vi "Signal Loop.vi"(8 "error in (no error)":errorcluster, 11 "CLI in":refnum<class "CLI.lvclass">) -> (0 "error out":errorcluster)   [LabVIEW 2017, in "CLI.lvclass"]
uses:
  CLI.lvclass
  CLI.lvclass/CLI.ctl
panel:
  # "Connector Pane"
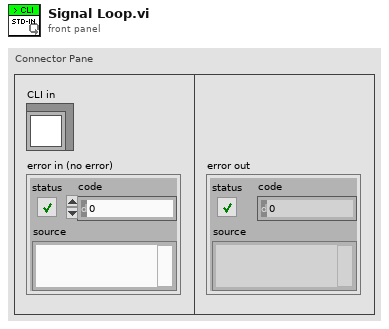
[diagram p1: front panel]
types:
  T1 = typedef "Events.ctl" = cluster{"STIN":refnum<user-event>, "SIGI":refnum<user-event>, "UnknownSignal":refnum<user-event>}
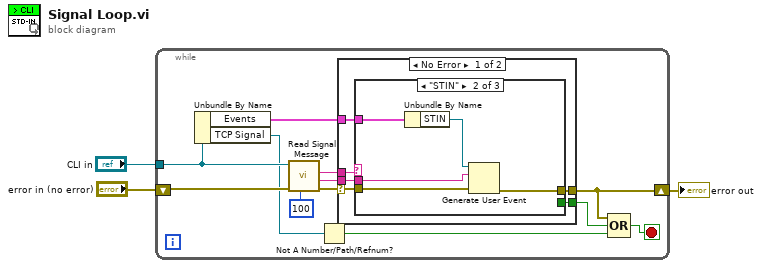
[diagram p0: block diagram]
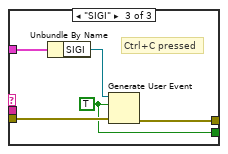
[diagram p3: hidden frame]
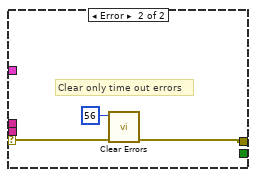
[diagram p4: hidden frame]
diagram:
  n1 = while {
    tunnel: "CLI in" -> [w10]
    shift-right: [w5] -> w1
    shift-left: "error in (no error)" -> [w15]
    stop <- w11 stop-if-true
    n2 = Unbundle By Name(w10) -> ("Events"=w7:T1, "TCP Signal"=w9:refnum<k5>)
    n3 = call "Read Signal Message.vi"("timeout ms (25000)"=100, "error in (no error)"=w15, "CLI in"=w10) -> ("error out"=w12:errorcluster, "Message Contents"=w13:string, "Message Type"=w14:string)  [unwired: 5 in, 1 out]
    n4 = Not A Number/Path/Refnum?(number/path/refnum=w9) -> (NaN/Path/Refnum?=w8:bool)
    n5 = case shown="No Error" w12 {
      selector: w12 -> [w19 w35]
      tunnel: w14 -> [w21 _]
      tunnel: w13 -> [w20 _]
      tunnel: w7 -> [w18 _]
      tunnel: [w17 w34] -> w5
      tunnel: [w16 _] -> w4
      frame No Error {
        n6 = case shown="\"STIN\"" w21 {
          tunnel: w18 -> [_ w23 w29]
          tunnel: w20 -> [_ w26 _]
          tunnel: w19 -> [w22 w25 w31]
          tunnel: [w22 w24 w30] -> w17
          tunnel: [_ _ w28] -> w16
          frame Default {
          }
          frame "STIN" {
            n7 = Unbundle By Name(w23) -> ("STIN"=w27:refnum<user-event>)
            n8 = Generate User Event(user event=w27, event data cluster=w26, error in=w25) -> (error out=w24:errorcluster)  [unwired: 1 in, 1 out]
          }
          frame "SIGI" {
            w28 = TRUE ("event data")
            # "Ctrl+C pressed"
            n9 = Unbundle By Name(w29) -> ("SIGI"=w32:refnum<user-event>)
            n10 = Generate User Event(user event=w32, event data cluster=w28, error in=w31) -> (error out=w30:errorcluster)  [unwired: 1 in, 1 out]
          }
        }
      }
      frame Error {
        # "Clear only time out errors"
        n11 = call <vilib>:"Clear Errors.vi"("error in (no error)"=w35, "specific error code to clear (0: all)"=56) -> ("error out"=w34:errorcluster)  [unwired: 4 in, 1 out]
      }
    }
    n12 = Compound Arithmetic op=OR(w5, w4, w8) -> (w11:bool)
  }
  "error out" <- w1
